vi "Get STL dimensions.vi"(0 "Stl Filenames":path[](array[path])) -> (1 "Limits":sgl[][](array[numeric]), 2 "Error out":errorcluster, 3 "stl Files":string[](array[string]))   [LabVIEW 2020]
panel:
  # "PN 21/11/17"
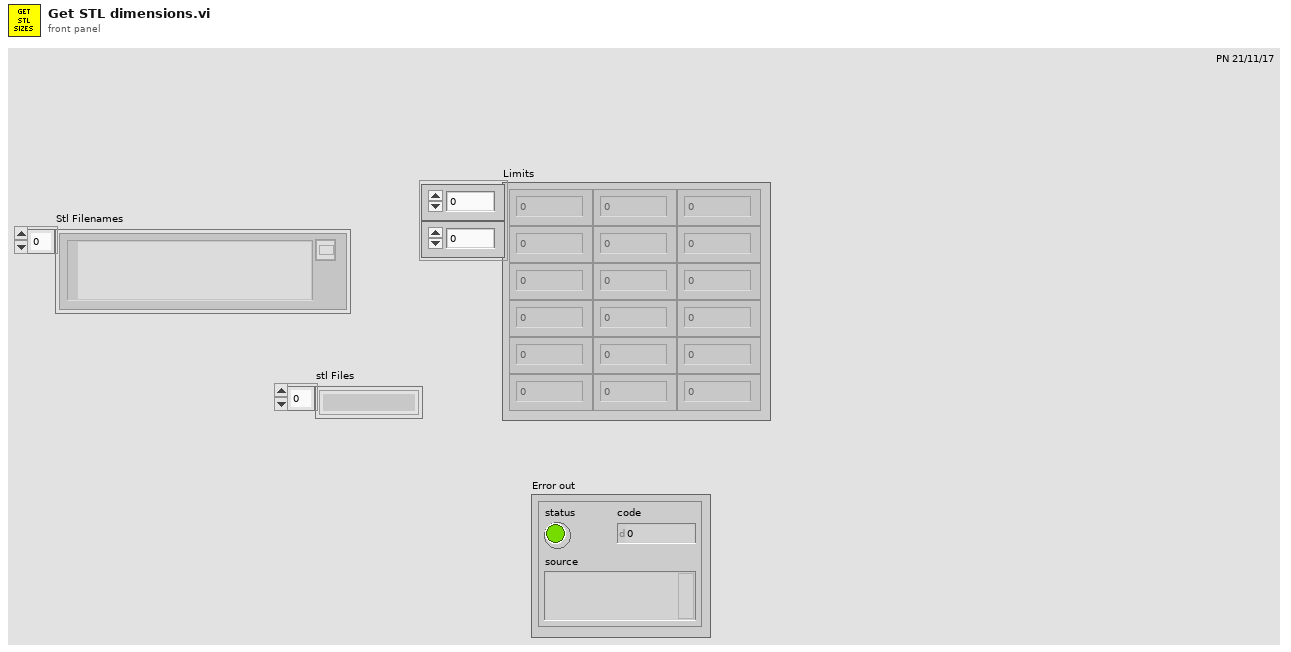
[diagram p1: front panel]
types:
  T1 = typedef "Triangle panel.ctl" = cluster{"V0":sgl[], "V1":sgl[], "V2":sgl[], "E0":sgl[], "E1":sgl[], "E2":sgl[], "n^":sgl[], "Pc":sgl[], "Gamma'":sgl, "V_transp.":sgl, "E0 link":i32, "E1 link":i32, "E2 link":i32}
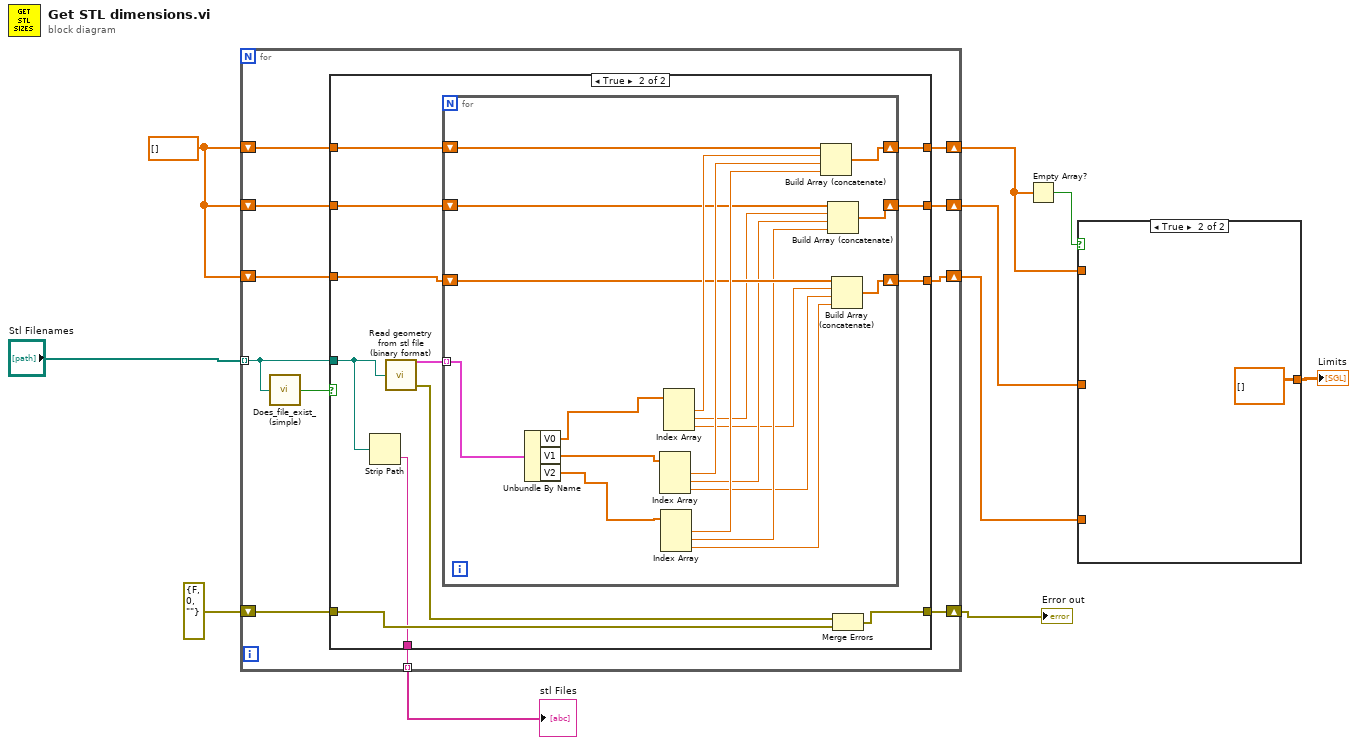
[diagram p0: block diagram]
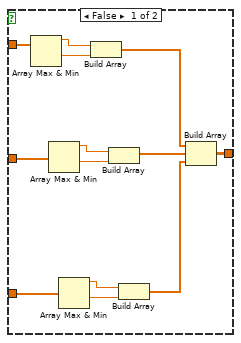
[diagram p2: hidden frame]
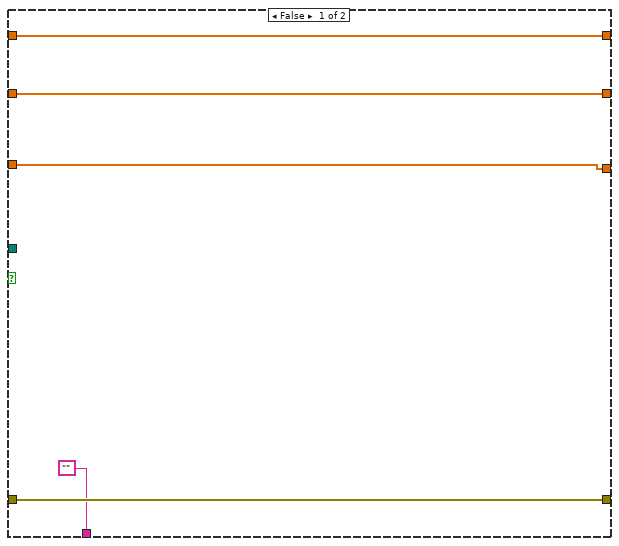
[diagram p3: hidden frame]
diagram:
  w9 = sgl[] []
  n1 = for {
    shift-right: [w16] -> w2
    shift-left: w9 -> [w19]
    shift-right: [w17] -> w7
    shift-left: w9 -> [w20]
    shift-right: [w18] -> w6
    shift-left: w9 -> [w21]
    tunnel: "Stl Filenames" -> [w13] mode=indexing
    shift-right: [w15] -> w4
    shift-left: errorcluster {"status"=FALSE, "code"=0, "source"=""} ("error IO") -> [w14]
    tunnel: [w11] -> w3 mode=indexing
    n2 = call "Does_file_exist_(simple).vi"("Pathname"=w13) -> ("exists?"=w12:bool)
    n3 = case shown="True" w12 {
      tunnel: w21 -> [w24 w37]
      tunnel: w20 -> [w25 w36]
      tunnel: w19 -> [w26 w35]
      tunnel: [w24 w34] -> w18
      tunnel: [w25 w33] -> w17
      tunnel: [w26 w32] -> w16
      tunnel: [w23 w30] -> w15
      tunnel: w14 -> [w23 w29]
      tunnel: w13 -> [_ w28]
      tunnel: ["" w27] -> w11
      frame False {
      }
      frame True {
        n4 = Strip Path(path=w28) -> (name=w27:string)  [unwired: 1 out]
        n5 = call "Read geometry from stl file (binary format).vi"("STL file path"=w28) -> ("Panel triangles array"=w38:T1[], "Error out"=w31:errorcluster)  [unwired: 1 out]
        n6 = for {
          tunnel: w38 -> [w57] mode=indexing
          shift-right: [w49] -> w32
          shift-left: w35 -> [w53]
          shift-right: [w48] -> w33
          shift-left: w36 -> [w47]
          shift-right: [w39] -> w34
          shift-left: w37 -> [w46]
          n7 = Unbundle By Name(w57) -> ("V0"=w54:sgl[], "V1"=w56:sgl[], "V2"=w55:sgl[])
          n8 = Index Array(array=w56) -> (element #1=w51:sgl, element #2=w44:sgl, element #3=w41:sgl)  [unwired: 3 in]
          n9 = Index Array(array=w55) -> (element #1=w50:sgl, element #2=w43:sgl, element #3=w40:sgl)  [unwired: 3 in]
          n10 = Index Array(array=w54) -> (element #1=w52:sgl, element #2=w45:sgl, element #3=w42:sgl)  [unwired: 3 in]
          n11 = Build Array (concatenate)(w53, w52, w51, w50) -> (w49:sgl[])
          n12 = Build Array (concatenate)(w47, w45, w44, w43) -> (w48:sgl[])
          n13 = Build Array (concatenate)(w46, w42, w41, w40) -> (w39:sgl[])
        }
        n14 = Merge Errors(w31, w29) -> (w30:errorcluster)
      }
    }
  }
  "Error out" <- w4
  "stl Files" <- w3
  n15 = Empty Array?(array=w2) -> (empty?=w1:bool)
  n16 = case shown="True" w1 {
    tunnel: [w70 sgl[][] []] -> w10
    tunnel: w7 -> [w60 _]
    tunnel: w6 -> [w59 _]
    tunnel: w2 -> [w58 _]
    frame False {
      n17 = Array Max & Min(array=w58) -> (max value=w69:sgl, min value=w68:sgl)  [unwired: 2 out]
      n18 = Array Max & Min(array=w60) -> (max value=w66:sgl, min value=w67:sgl)  [unwired: 2 out]
      n19 = Array Max & Min(array=w59) -> (max value=w65:sgl, min value=w64:sgl)  [unwired: 2 out]
      n20 = Build Array(w69, w68) -> (w61:sgl[])
      n21 = Build Array(w66, w67) -> (w62:sgl[])
      n22 = Build Array(w65, w64) -> (w63:sgl[])
      n23 = Build Array(w61, w62, w63) -> (w70:sgl[][])
    }
    frame True {
    }
  }
  "Limits" <- w10
